vi "deserialize.vi"(8 "error in":errorcluster, 10 "serialized form":string, 11 "configuration in":refnum<class "NISE_CEF_serializable configuration.lvclass">) -> (0 "error out":errorcluster, 3 "configuration out":refnum<class "NISE_CEF_serializable configuration.lvclass">)   [LabVIEW 2013, in "NISE_CEF_serializable configuration.lvclass"]
uses:
  NISE_CEF_serializable configuration.lvclass
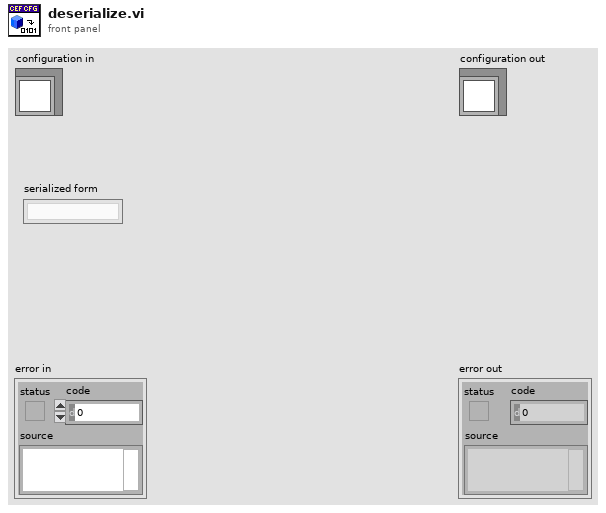
[diagram p1: front panel]
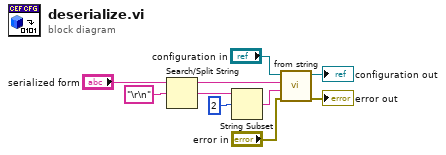
[diagram p0: block diagram]
diagram:
  n1 = Search/Split String(string="serialized form", search string/char (-)="\r\n" ("concatenated string")) -> (substring before match=w1:string, match + rest of string=w4:string)  [unwired: 1 in, 1 out]
  n2 = String Subset(string=w4, offset (0)=2) -> (substring=w2:string)  [unwired: 1 in]
  n3 = call-dynamic "from string.vi"("error in"="error in", "data"=w2, "version"=w1, "configuration in"="configuration in") -> ("error out"=→"error out":errorcluster, "configuration out"=→"configuration out":refnum<class "NISE_CEF_serializable configuration.lvclass">)  [unwired: 6 in]
